vi "ConvertInputsTo64PinArray.vi"(11 "Inputs":T2[](array[typedef])) -> (3 "64-Pin Array":T1(array[cluster]))   [LabVIEW 2012, in "Virtual-PGA.lvlib"]
uses:
  Public/Controls/Input.ctl
  Virtual-PGA.lvlib
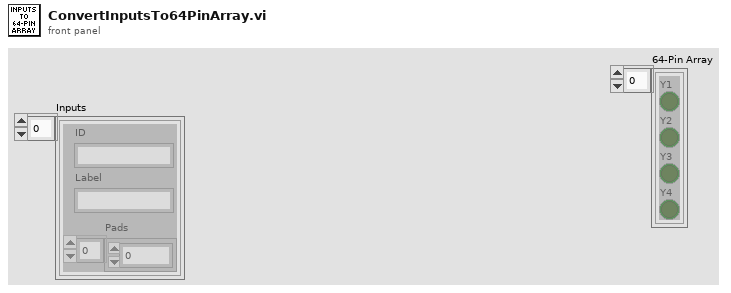
[diagram p1: front panel]
types:
  T1 = cluster{"Y1":bool, "Y2":bool, "Y3":bool, "Y4":bool}[]
  T2 = typedef "Virtual-PGA.lvlib/Input.ctl" = cluster{"ID":string, "Label":string, "Pads":u32[]}
  T3 = cluster{"Y1":bool, "Y2":bool, "Y3":bool, "Y4":bool}
  T4 = cluster{"Pad[0]":bool, "Pad[1]":bool, "Pad[2]":bool, "Pad[3]":bool}
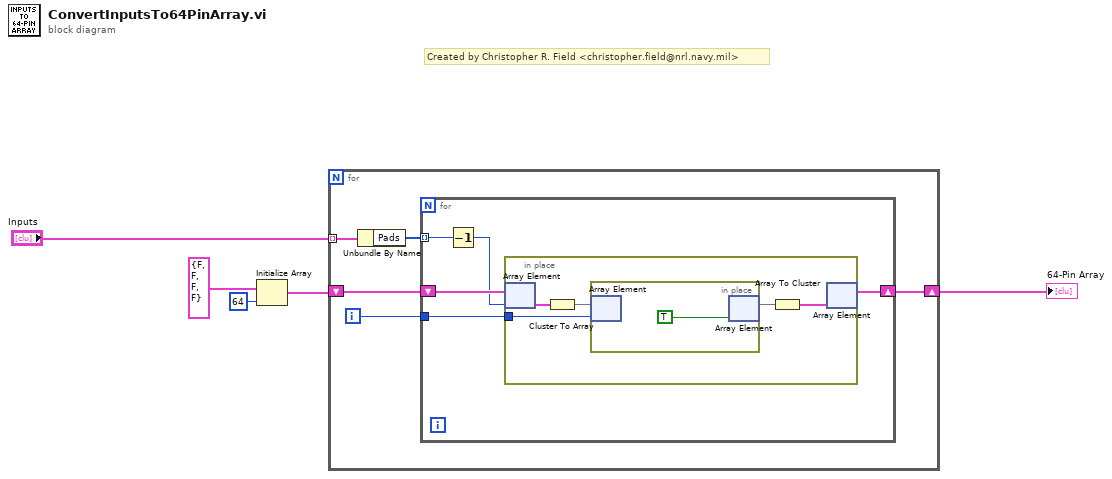
[diagram p0: block diagram]
diagram:
  # "Created by Christopher R. Field <christopher.field@nrl.navy.mil>"
  n1 = Initialize Array(T3 {"Y1"=FALSE, "Y2"=FALSE, "Y3"=FALSE, "Y4"=FALSE} ("Pad"), 64 ("dimension size")) -> (w1:T1)
  n2 = for {
    tunnel: "Inputs" -> [w10] mode=indexing
    shift-right: [w6] -> w4
    shift-left: w1 -> [w8]
    i -> [w7]
    n3 = Unbundle By Name(w10) -> ("Pads"=w9:u32[])
    n4 = for {
      tunnel: w9 -> [w15] mode=indexing
      tunnel: w7 -> [w12]
      shift-right: [w11] -> w6
      shift-left: w8 -> [w14]
      n5 = Decrement(x=w15) -> (x-1=w13:u32)
      n6 = in-place {
        in-place-border: w12 -> [w18]
        n7 = in-place-array #1(w14, w13) -> (w20:T3)
        n8 = Cluster To Array(cluster=w20) -> (array=w19:bool[])
        n9 = in-place {
          n10 = in-place-array #2(w19, w18) -> ()  [unwired: 1 out]
          n11 = in-place-array #2(TRUE ("new element/subarray")) -> (w17:bool[])  [unwired: 1 out]
        }
        n12 = Array To Cluster(array=w17) -> (cluster=w16:T4)
        n13 = in-place-array #1(w16) -> (w11:T1)  [unwired: 1 out]
      }
    }
  }
  "64-Pin Array" <- w4
